vi "Phasics process raw.vi"(8 "error in (no error)":errorcluster, 9 "Image in":i16[][](array[numeric]), 11 "Phasics Camera in":refnum<class "Phasics Camera.lvclass">) -> (0 "error out":errorcluster, 3 "Phasics Camera out":refnum<class "Phasics Camera.lvclass">, 4 "Phase out":sgl[][](array[numeric]), 5 "Intensity out":sgl[][](array[numeric]))   [LabVIEW 2013, in "Phasics Camera.lvclass"]
uses:
  Phasics Camera.lvclass
  Phasics Camera.lvclass/Phasics Camera.ctl
panel:
  out "Phase MaxMin":sgl[](array[numeric])
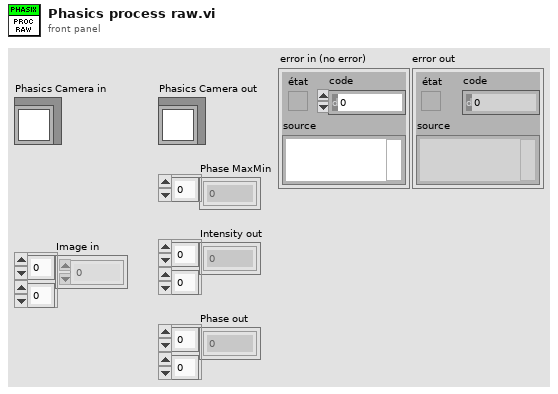
[diagram p1: front panel]
types:
  T1 = typedef "Refnum SDKSID4 session.ctl" = refnum<k1>
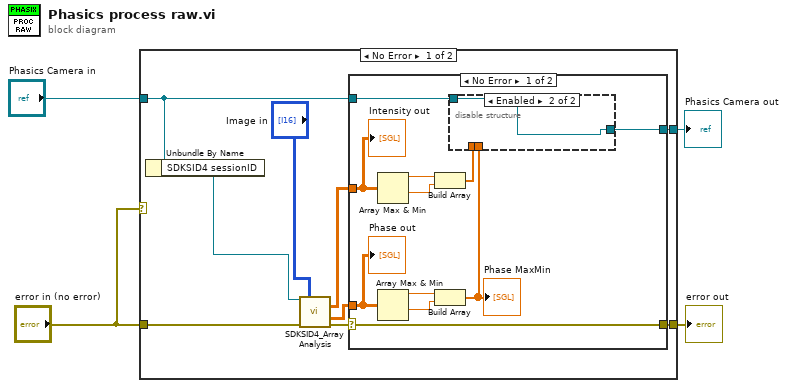
[diagram p0: block diagram]
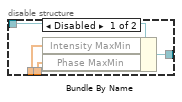
[diagram p2: hidden frame]
diagram:
  n1 = case shown="No Error" "error in (no error)" {
    tunnel: [w13 w32] -> w4
    tunnel: "Phasics Camera in" -> [w6 w32]
    tunnel: "error in (no error)" -> [w9 w33]
    tunnel: [w7 w33] -> w2
    frame No Error {
      n2 = Unbundle By Name(w6) -> ("SDKSID4 sessionID"=w5:T1)
      n3 = call "SDKSID4_Array Analysis.vi"("SDKSID4 session In"=w5, "Interferogram in (ArrayI16)"="Image in", "error in (no error)"=w9) -> ("Intensity out"=w11:sgl[][], "Phase out"=w10:sgl[][], "error out"=w8:errorcluster)  [unwired: 8 in, 2 out]
      n4 = case shown="No Error" w8 {
        selector: w8 -> [w14 w31]
        tunnel: [w24 w30] -> w13
        tunnel: w6 -> [w23 w30]
        tunnel: w11 -> [w16 _]
        tunnel: w10 -> [w15 _]
        tunnel: [w14 w31] -> w7
        frame No Error {
          n5 = Array Max & Min(array=w16) -> (max value=w21:sgl, min value=w22:sgl)  [unwired: 2 out]
          n6 = Array Max & Min(array=w15) -> (max value=w19:sgl, min value=w20:sgl)  [unwired: 2 out]
          n7 = Build Array(w21, w22) -> (w18:sgl[])
          n8 = Build Array(w19, w20) -> (w17:sgl[])
          "Phase MaxMin" <- w17
          n9 = disable-structure shown="Enabled" {
            disable-tunnel: [w28 w29] -> w24
            disable-tunnel: w23 -> [w27 w29]
            disable-tunnel: w18 -> [w26 _]
            disable-tunnel: w17 -> [w25 _]
            frame Disabled {
              n10 = Bundle By Name(cluster=w27, "Intensity MaxMin"=w26, "Phase MaxMin"=w25) -> (w28:refnum<class "Phasics Camera.lvclass">)
            }
            frame Enabled {
            }
          }
          "Intensity out" <- w16
          "Phase out" <- w15
        }
        frame Error {
        }
      }
    }
    frame Error {
    }
  }
  "Phasics Camera out" <- w4
  "error out" <- w2
